vi "Pass if Number of Test Suite Results.vi"(8 "error in (no error)":errorcluster, 9 "Results":T1[](array[typedef]), 10 "Remaining Results":i32, 11 "LUnit Test Suite Tests in":refnum<class "LUnit Test Suite Tests.lvclass">) -> (0 "error out":errorcluster, 3 "LUnit Test Suite Tests out":refnum<class "LUnit Test Suite Tests.lvclass">)   [LabVIEW 2020, in "LUnit Test Suite Tests.lvclass"]
uses:
  LUnit Test Suite Tests.lvclass
  LUnit Test Suite Tests.lvclass/LUnit Test Suite Tests.ctl
  f642ace2-917c-459c-805b-ee2307aec75e.vi
  source/Core/Result/Type.ctl
  source/Core/Result/Result.lvlib
  source/Core/Result/Status.ctl
  source/Core/Result/Result.ctl
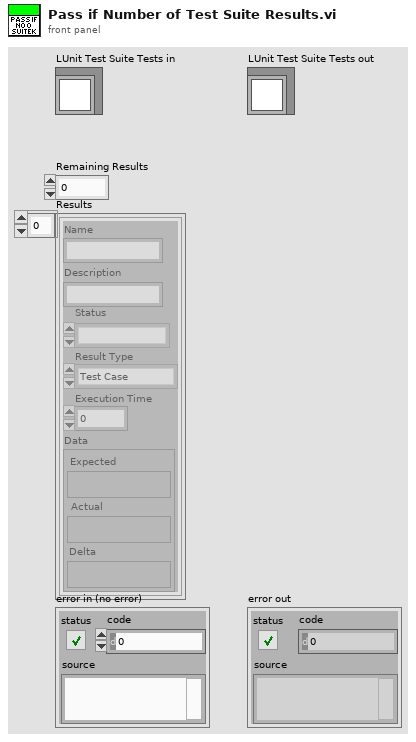
[diagram p1: front panel]
types:
  T1 = typedef "Result.lvlib/Result.ctl" = cluster{"Name":string, "Description":string, "Status":T2, "Result Type":T3, "Execution Time":dbl, "Data":cluster{"Expected":variant, "Actual":variant, "Delta":variant}}
  T2 = typedef "Result.lvlib/Status.ctl" = enum16{"", "Passed", "Failed", "Error", "Skipped", "Setup Error", "Broken", "Teardown Error"}
  T3 = typedef "Result.lvlib/Type.ctl" = enum16{"Test Case", "Test Suite", "Test Run", "Pass", "Fail", "Skip", "Pass if", "Fail if", "Pass if Error", "Fail if Error", "Pass if Equal", "Fail if Equal"}
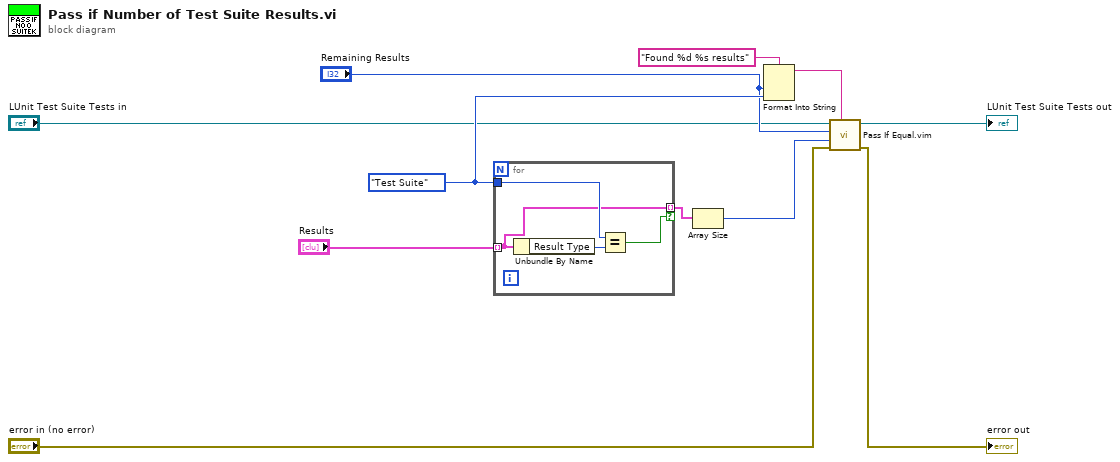
[diagram p0: block diagram]
diagram:
  w10 = Type."Test Suite" ("x")
  n1 = for {
    tunnel: "Results" -> [w13] mode=indexing
    tunnel: w10 -> [w14]
    tunnel: [w13] -> w6 mode=indexing if=w12
    n2 = Unbundle By Name(w13) -> ("Result Type"=w15:T3)
    n3 = Equal?(x=w14, y=w15) -> (x = y?=w12:bool)
  }
  n4 = Array Size(array=w6) -> (size(s)=w7:i32)
  n5 = Format Into String(format string="Found %d %s results", "Remaining Results", w10) -> (resulting string=w11:string)  [unwired: 2 in, 1 out]
  n6 = call "Pass If Equal.vim"("Description"=w11, "error in (no error)"="error in (no error)", "Actual"=w7, "Expected"="Remaining Results", "LUnit Test Case In"="LUnit Test Suite Tests in") -> ("error out"=→"error out":errorcluster, "LUnit Test Case Out"=→"LUnit Test Suite Tests out":refnum<class "LUnit Test Suite Tests.lvclass">)  [unwired: 5 in]
